vi "Button.vi"(11 "Button In":bool) -> (3 "Button Pressed?":bool)   [LabVIEW 2019]
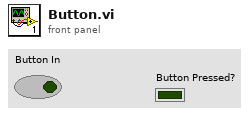
[diagram p1: front panel]
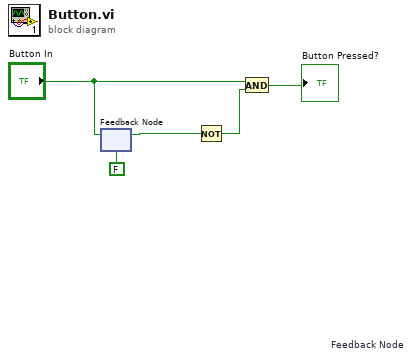
[diagram p0: block diagram]
diagram:
  n1 = feedback-in #1("Button In") -> ()
  n2 = feedback #1 "Feedback Node"(FALSE ("Button In")) -> (w3:bool)
  n3 = Not(x=w3) -> (.not. x?=w4:bool)
  n4 = And(x="Button In", y=w4) -> (x .and. y?=→"Button Pressed?":bool)
